vi "Send Output.vi"(8 "error in (no error)":errorcluster, 11 "57XX in":refnum<class "57XX.lvclass">) -> (0 "error out":errorcluster, 3 "57XX out":refnum<class "57XX.lvclass">)   [LabVIEW 2019, in "57XX.lvlib" / "57XX.lvclass"]
uses:
  Library/57XX.lvclass
  C:/Users/Public/Documents/Development/builds/Instruments/PowerSupply.lvlibp/Library/PowerSupply.lvclass
  Library/57XX.lvclass/57XX.ctl
  Accessors/Read Local Resource.vi
  Accessors/Write Local Resource.vi
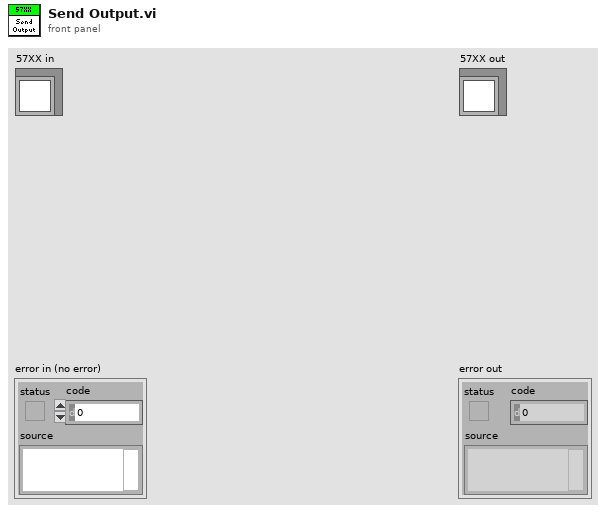
[diagram p1: front panel]
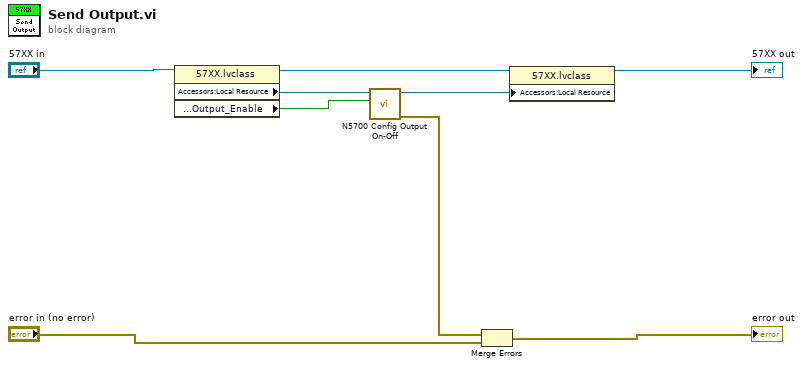
[diagram p0: block diagram]
diagram:
  n1 = property class="57XX.lvclass"(reference="57XX in") -> (reference out=w6:refnum<class "57XX.lvclass">, "Accessors:Local Resource"=w5:refnum<visa-resource-name>, "Accessors:Setting:Output_Enable"=w3:bool)  [unwired: 1 in, 1 out]
  n2 = call <instrlib>:"N5700 Config Output On-Off.vi"("Output ON"=w3, "VISA"=w5) -> ("error out"=w9:errorcluster, "VISA out"=w4:refnum<visa-resource-name>)  [unwired: 5 in]
  n3 = Merge Errors(w9, "error in (no error)") -> (→"error out":errorcluster)
  n4 = property class="57XX.lvclass"(reference=w6, "Accessors:Local Resource"=w4) -> (reference out=→"57XX out":refnum<class "57XX.lvclass">)  [unwired: 1 in, 1 out]
